vi "Load_Template_Globals.vi"(1 "Channel Names":string[](array[string]), 2 "Template-read":path) -> (0 "Valid Template File?":bool)   [LabVIEW 2015]
uses:
  Controls/Global_mode.ctl
  Results_plotter_Global.vi
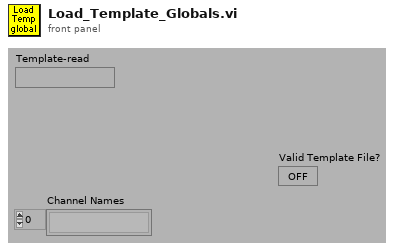
[diagram p1: front panel]
types:
  T1 = typedef "Global_mode.ctl" = enum16{"Read Global", "Load Global From File", "Write Global to File"}
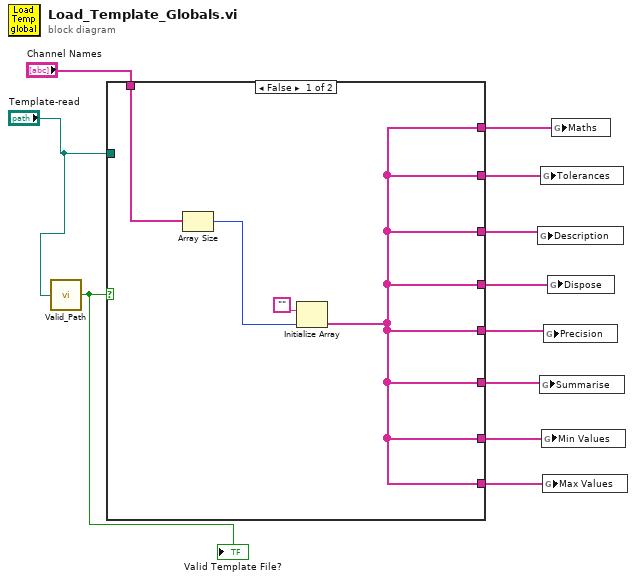
[diagram p0: block diagram]
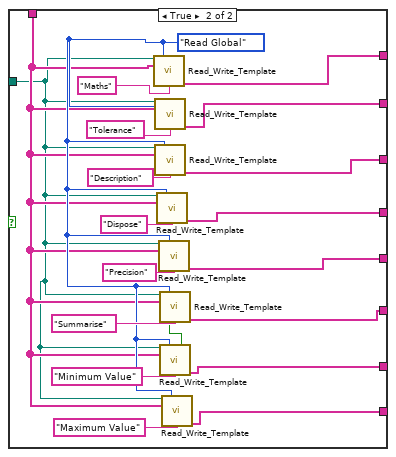
[diagram p2: hidden frame]
diagram:
  n1 = call "Valid_Path.vi"("Filename"="Template-read") -> ("Valid Path?"=w4:bool)
  "Valid Template File?" <- w4
  n2 = case shown="False" w4 {
    tunnel: "Template-read" -> [_ w18]
    tunnel: "Channel Names" -> [w14 w19]
    tunnel: [w12 w30] -> w7
    tunnel: [w12 w29] -> w8
    tunnel: [w12 w28] -> w9
    tunnel: [w12 w27] -> w10
    tunnel: [w12 w26] -> w11
    tunnel: [w12 w24] -> w3
    tunnel: [w12 w17] -> w2
    tunnel: [w12 w16] -> w1
    frame False {
      n3 = Array Size(array=w14) -> (size(s)=w13:i32)
      n4 = Initialize Array("", w13) -> (w12:string[])
    }
    frame True {
      w20 = Global_mode."Read Global" ("Mode")
      n5 = call "Read_Write_Template.vi"("Template File"=w18, "Mode"=w20, "Channel names In"=w19, "Data type"="Maths") -> ("1D Info Out"=w24:string[])  [unwired: 4 in, 7 out]
      n6 = call "Read_Write_Template.vi"("Template File"=w18, "Mode"=w20, "Channel names In"=w19, "Data type"="Tolerance") -> ("1D Info Out"=w26:string[])  [unwired: 4 in, 7 out]
      n7 = call "Read_Write_Template.vi"("Template File"=w18, "Mode"=w20, "Channel names In"=w19, "Data type"="Description") -> ("1D Info Out"=w27:string[])  [unwired: 4 in, 7 out]
      n8 = call "Read_Write_Template.vi"("Template File"=w18, "Mode"=w20, "Channel names In"=w19, "Data type"="Dispose") -> ("1D Info Out"=w28:string[])  [unwired: 4 in, 7 out]
      n9 = call "Read_Write_Template.vi"("Template File"=w18, "Mode"=w20, "Channel names In"=w19, "Data type"="Precision") -> ("1D Info Out"=w29:string[])  [unwired: 4 in, 7 out]
      n10 = call "Read_Write_Template.vi"("Template File"=w18, "Mode"=w20, "Channel names In"=w19, "Data type"="Minimum Value") -> ("Freshly Loaded?"=w22:bool, "1D Info Out"=w17:string[])  [unwired: 4 in, 6 out]
      n11 = call "Read_Write_Template.vi"("Template File"=w18, "Mode"=w20, "Channel names In"=w19, "Save file"=w22, "Data type"="Summarise") -> ("1D Info Out"=w30:string[])  [unwired: 3 in, 7 out]
      n12 = call "Read_Write_Template.vi"("Template File"=w18, "Mode"=w20, "Channel names In"=w19, "Data type"="Maximum Value") -> ("1D Info Out"=w16:string[])  [unwired: 4 in, 7 out]
    }
  }
  n13 = global write "Results_plotter_Global.vi" "Description"(w10) -> ()
  n14 = global write "Results_plotter_Global.vi" "Summarise"(w7) -> ()
  n15 = global write "Results_plotter_Global.vi" "Tolerances"(w11) -> ()
  n16 = global write "Results_plotter_Global.vi" "Min Values"(w2) -> ()
  n17 = global write "Results_plotter_Global.vi" "Max Values"(w1) -> ()
  n18 = global write "Results_plotter_Global.vi" "Precision"(w8) -> ()
  n19 = global write "Results_plotter_Global.vi" "Dispose"(w9) -> ()
  n20 = global write "Results_plotter_Global.vi" "Maths"(w3) -> ()
